vi "Julabo_Display_Values_subVI.vi"(8 "error in (no error)":errorcluster, 10 "Setpointindex":enum16{"Setpoint 1", "Setpoint 2", "Setpoint 3"}(ring), 11 "VISA Refnum in":refnum<visa-resource-name>) -> (0 "error out":errorcluster, 1 "Safety Temp":dbl, 2 "Excess Temp Protection":dbl, 3 "VISA Refnum out":refnum<visa-resource-name>, 4 "Power":i8(slide) scale=-100.0..100.0, 5 "Internal Temp":dbl format="%.2f", 6 "External Temp":dbl format="%.2f", 7 "Diagram":T1(graph))   [LabVIEW 2015, in "JULABO DeviceDriver.lvlib"]
uses:
  <instrlib>/JULABO DeviceDriver/JULABO DeviceDriver.lvlib
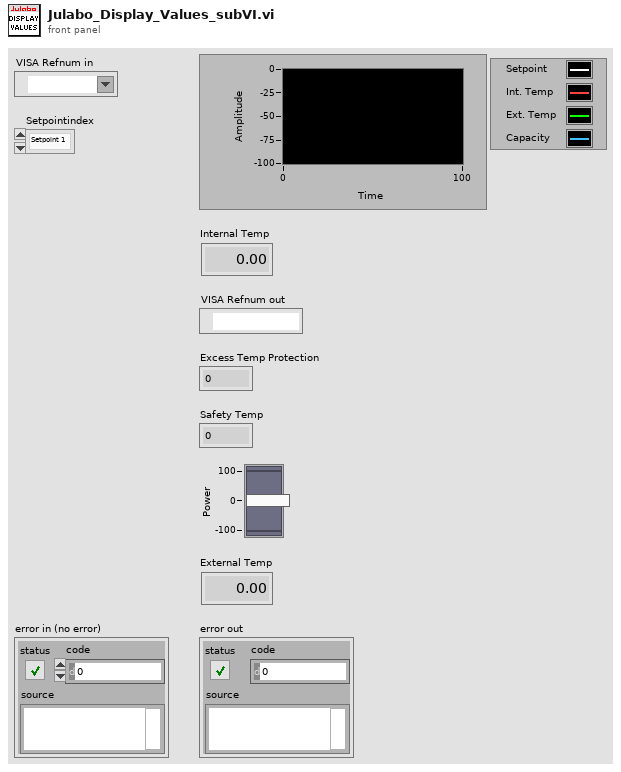
[diagram p1: front panel]
types:
  T1 = cluster{"Setpoint (out)":dbl, "InternalTemp (out)":dbl, "ExternalTemp (out)":dbl, "Capacity (out)":i8}
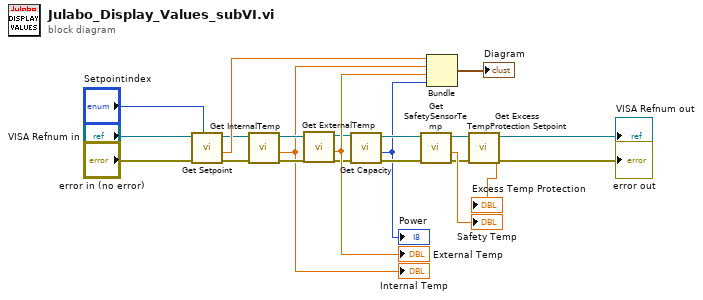
[diagram p0: block diagram]
diagram:
  n1 = call <instrlib>:"Get Setpoint.vi"("Setpointindex"="Setpointindex", "error in (no error)"="error in (no error)", "VISA resource name"="VISA Refnum in") -> ("error out"=w1:errorcluster, "Setpoint (out)"=w7:dbl, "VISA resource name out"=w2:refnum<visa-resource-name>)  [unwired: 6 in]
  n2 = call <instrlib>:"Get InternalTemp.vi"("error in (no error)"=w1, "VISA resource name"=w2) -> ("error out"=w9:errorcluster, "InternalTemp (out)"=w4:dbl, "VISA resource name out"=w8:refnum<visa-resource-name>)  [unwired: 7 in]
  "Internal Temp" <- w4
  n3 = call <instrlib>:"Get ExternalTemp.vi"("error in (no error)"=w9, "VISA resource name"=w8) -> ("error out"=w11:errorcluster, "ExternalTemp (out)"=w13:dbl, "VISA resource name out"=w10:refnum<visa-resource-name>)  [unwired: 6 in, 1 out]
  "External Temp" <- w13
  n4 = call <instrlib>:"Get Capacity.vi"("error in (no error)"=w11, "VISA resource name"=w10) -> ("error out"=w19:errorcluster, "Capacity (out)"=w12:i8, "VISA resource name out"=w14:refnum<visa-resource-name>)  [unwired: 7 in]
  "Power" <- w12
  n5 = call <instrlib>:"Get SafetySensorTemp.vi"("error in (no error)"=w19, "VISA resource name"=w14) -> ("error out"=w18:errorcluster, "Safetytemp (out)"=→"Safety Temp":dbl, "VISA resource name out"=w15:refnum<visa-resource-name>)  [unwired: 7 in]
  n6 = Bundle("Setpoint (out)"=w7, "InternalTemp (out)"=w4, "ExternalTemp (out)"=w13, "Capacity (out)"=w12) -> (→"Diagram":T1)  [unwired: 1 in]
  n7 = call <instrlib>:"Get Excess TempProtection Setpoint.vi"("error in (no error)"=w18, "VISA resource name"=w15) -> ("error out"=→"error out":errorcluster, "ExcessTempProtection(out)"=→"Excess Temp Protection":dbl, "VISA resource name out"=→"VISA Refnum out":refnum<visa-resource-name>)  [unwired: 7 in]
